vi "Pre Launch Init.vi"(11 "MainPage in":refnum<class "MainPage.lvclass"> caption="操作者输入") -> (0 "error out":errorcluster caption="错误输出", 3 "MainPage out":refnum<class "MainPage.lvclass"> caption="操作者输出")   [LabVIEW 2019, in "MainPage.lvlib" / "MainPage.lvclass"]
doc: "(<B>文件名</B>: Actor Framework.lvlib:Actor.lvclass:Pre Launch Init.vi)\n\n定义启动嵌套操作者方法被调用之后、操作者核心方法开始运行之前的操作。\n\n默认情况下，该方法不执行任何操作。子孙类重写该方法定义具体的操作。"
uses:
  MainPage.lvclass
  <vilib>/ActorFramework/Actor/Actor.lvclass
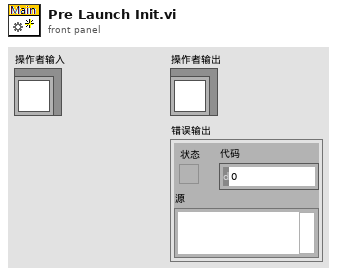
[diagram p1: front panel]
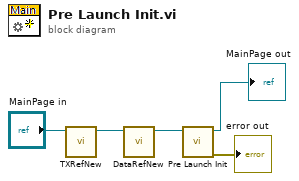
[diagram p0: block diagram]
diagram:
  n1 = call-dynamic "TXRefNew.vi"("MainPage 输入"="MainPage in") -> ("MainPage 输出"=w2:refnum<class "MainPage.lvclass">)  [unwired: 8 in, 2 out]
  n2 = call-dynamic "DataRefNew.vi"("MainPage 输入"=w2) -> ("MainPage 输出"=w1:refnum<class "MainPage.lvclass">)  [unwired: 8 in, 2 out]
  n3 = call-parent "Pre Launch Init.vi"("Actor in"=w1) -> ("error out"=→"error out":errorcluster, "Actor out"=→"MainPage out":refnum<class "MainPage.lvclass">)  [unwired: 9 in]
